vi "nanostage-close.vi"(1 "All conn. axes":string[](array[string])) -> (0 "error out":errorcluster)   [LabVIEW 2017]
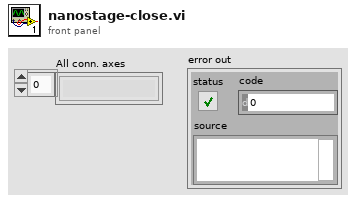
[diagram p1: front panel]
diagram:
  n1 = flat-sequence {
    tunnel: [w7] -> w6
    tunnel: w1 -> [w8]
    tunnel: [w10] -> w3
    tunnel: w6 -> [w11]
    tunnel: w1 -> [w12]
    tunnel: w3 -> [w29]
    tunnel: w1 -> [w26]
    tunnel: [w25] -> w2
    tunnel: [w31] -> w5
    tunnel: w2 -> [w32]
    tunnel: w1 -> [w30]
    tunnel: w5 -> [w37]
    tunnel: [w36] -> w4
    frame #0 {
      # "move to 0µm"
      n2 = call "nanostage-set.vi"("setValues"=dbl[] [], "Axes to move"=w8) -> ("error out"=w7:errorcluster)  [unwired: 1 in, 2 out]
    }
    frame #1 {
      # "check if moving completed"
      n3 = while {
        tunnel: w12 -> [w17]
        tunnel: w11 -> [w16]
        tunnel: [w14] -> w10
        stop <- w13 continue-if-true
        n4 = flat-sequence {
          tunnel: w16 -> [w18]
          tunnel: [w18] -> w15
          tunnel: w17 -> [w24]
          tunnel: w15 -> [w22]
          tunnel: [w21] -> w14
          tunnel: [w20] -> w13
          frame #0 {
            # "on target < 100ms"
            n5 = Wait (ms)(milliseconds to wait=u32 100) -> ()  [unwired: 1 out]
          }
          frame #1 {
            n6 = call "nanostage-check.vi"("error in"=w22, "axis set values"=dbl[] [], "Axes to move"=w24) -> ("error out"=w21:errorcluster, "moving"=w20:bool)  [unwired: 1 in, 2 out]
          }
        }
      }
    }
    frame #2 {
      # "servo loop off"
      n7 = call "SVO.vi"("System no."=1, "Axes to command"=w26, "Servo mode"=bool[] [FALSE, FALSE, FALSE], "error in"=w29) -> ("error out"=w25:errorcluster)  [unwired: 15 in]
    }
    frame #3 {
      # "analog 0V"
      n8 = call "SVA.vi"("System no."=1, "Axes to move"=w30, "PZT voltage"=dbl[] [0.0, 0.0, 0.0], "No.of digits"=i16 3, "error in"=w32) -> ("error out"=w31:errorcluster)  [unwired: 14 in]
    }
    frame #4 {
      n9 = call "Close connection if open.vi"("System no."=1, "error in"=w37) -> ("error out"=w36:errorcluster)  [unwired: 16 in, 1 out]
    }
  }
  n10 = local read "All conn. axes"() -> (w1:string[])
  "error out" <- w4
